vi "XNET CAN Signal Logger - MultiPorts.vi"() -> ()   [LabVIEW 2021, in "XNET-CAN-Signal-Logger.lvlib"]
uses:
  XNET-CAN-Signal-Logger.lvlib
  Typedef/Def-CAN Port Configuration.ctl
  Typedef/Def-Data Queue Ref.ctl
  Typedef/Def-Data Queue Type.ctl
  SubVIs/Global Variables.vi
  <resource>/objmgr/xnet.rc
panel:
  out "State:":string
  in  "Tab Control":enum32{"Analog Input", "CAN"}(tab)=enum."CAN"
  in  "CAN Configurations":T1[](array[typedef]) {"Sample Rate (Hz)" format="%#_13g"}
  in  "Stop Logging":bool
  out "Monitor.SignalUnits":string[](array[string])
  out "Monitor.SignalValues":dbl[](array[numeric])
  in  "Monitor.SignalNames":string[](array[combo])
  out "# elements in queue:":i32
  in  "Start Logging":bool
  out "Preview:":string
  in  "Log file name":string="LogFile_{Year}-{Month}-{Day}-{Hour}-{Minute}-{Second}.tdms"
  in  "Log file folder":path=path "C:/Users/NI/Desktop/Data"
  in  "Exit":bool
  # "Configuration"
  # "Signals to Monitor"
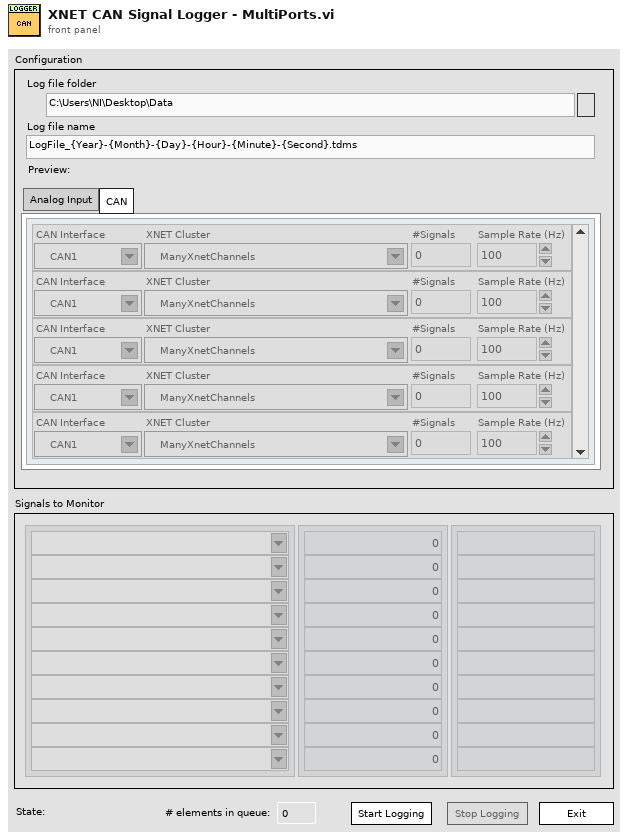
[diagram p1: front panel]
types:
  T1 = typedef "XNET-CAN-Signal-Logger.lvlib/Def-CAN Port Configuration.ctl" = cluster{"CAN Interface":refnum<k21>, "XNET Cluster":refnum<k21>, "#Signals":i32, "Sample Rate (Hz)":dbl}
  T2 = enum32{"Invalid", "Standard", "Closed", "Hidden", "Minimized", "Maximized"}
  T3 = enum32{"invalid app kind", "Development System", "Run Time System", "Student Edition", "Embedded LabVIEW", "Evaluation", "Custom"}
  T4 = enum8{"Enabled", "Disabled", "Disabled and Grayed Out"}
  T5 = typedef "XNET-CAN-Signal-Logger.lvlib/Def-Data Queue Type.ctl" = cluster{"PackageID":i32, "Data":waveform(dbl)[]}
  T6 = typedef "XNET-CAN-Signal-Logger.lvlib/Def-Data Queue Ref.ctl" = refnum<queue>
  T7 = cluster{"Core":cluster{"Current VI Reference":refnum<vi>, "Close Panel on Exit?":bool}, "Logging State":enum16{"Configure", "Logging"}, "LogFilePath":path, "CAN Configurations":refnum<vi>, "Data Queue Ref":T6, "Error Queue Ref":refnum<queue>, "Monitor.SignalNames":string[], "Monitor.SignalUnits":string[]}
  T8 = cluster{"Current VI Reference":refnum<vi>, "Close Panel on Exit?":bool}
  T9 = typedef "Def-CAN Port Configuration.ctl" = cluster{"CAN Interface":refnum<k21>, "XNET Cluster":refnum<k21>, "#Signals":i32, "Sample Rate (Hz)":dbl}
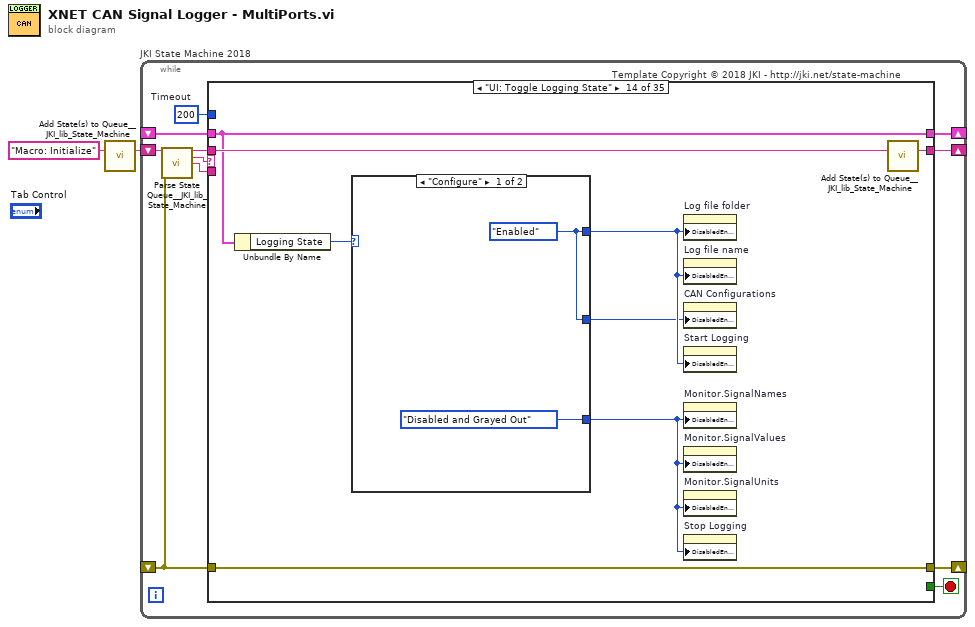
[diagram p0: block diagram]
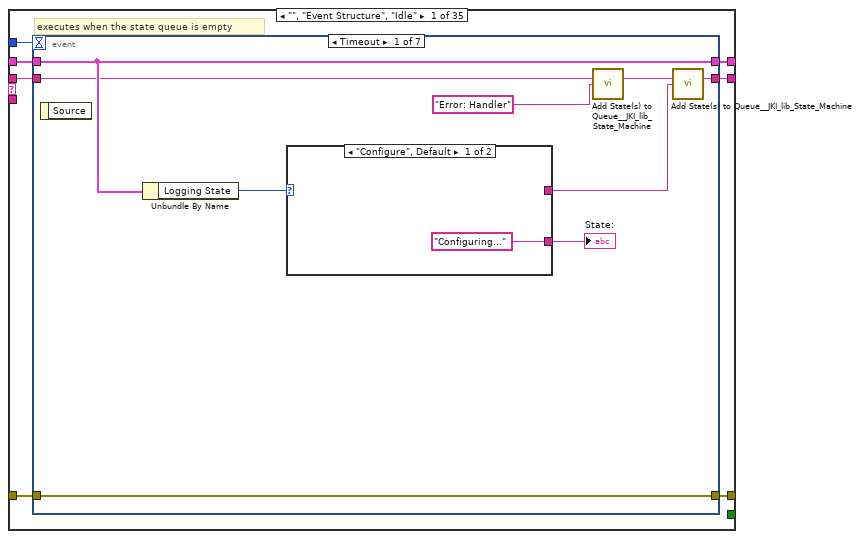
[diagram p2: hidden frame]
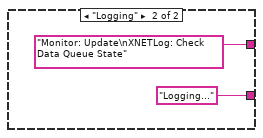
[diagram p3: hidden frame]
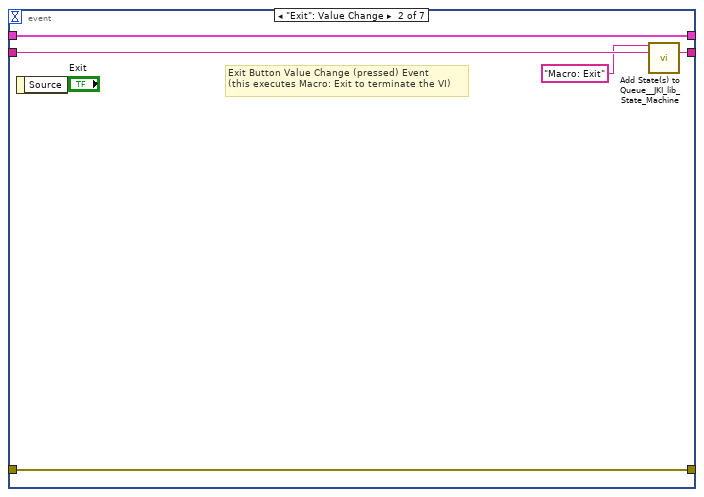
[diagram p4: hidden frame]
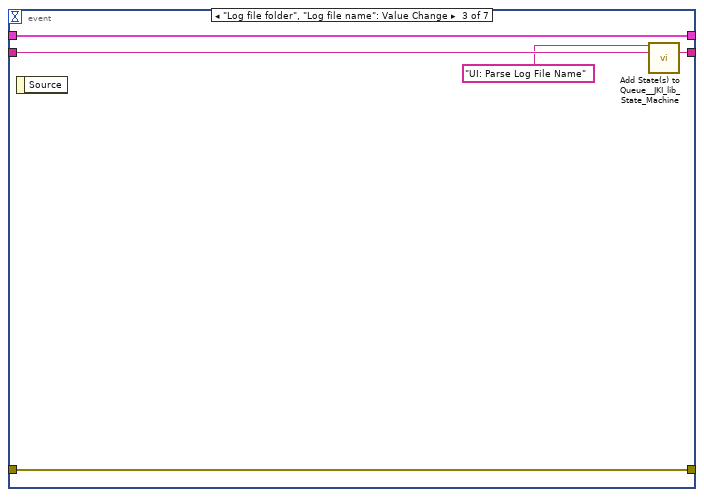
[diagram p5: hidden frame]
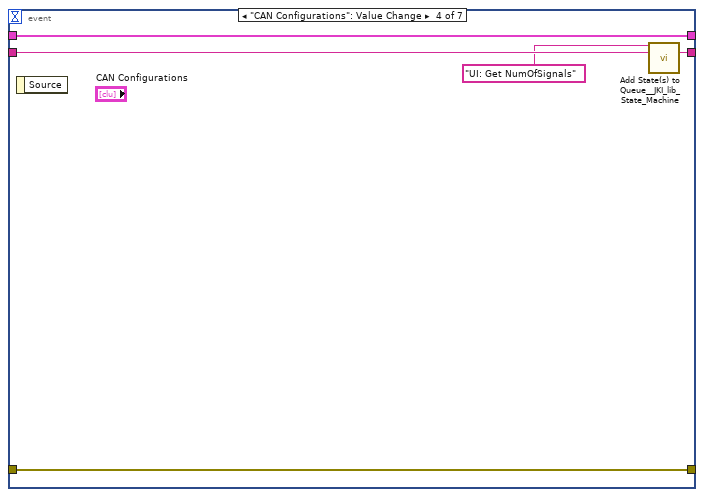
[diagram p6: hidden frame]
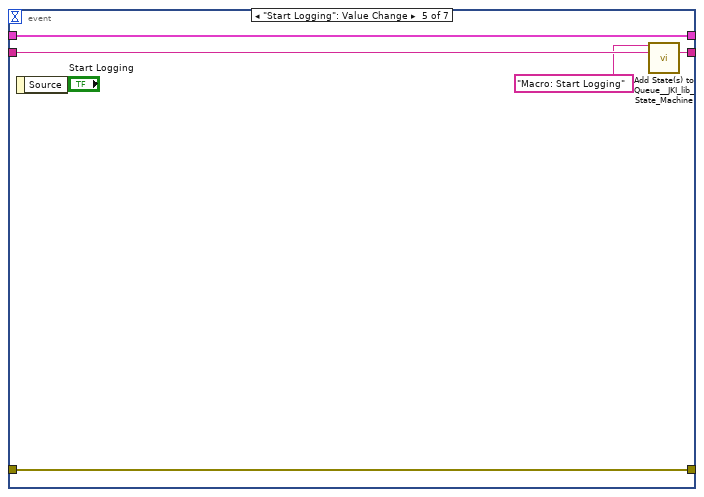
[diagram p7: hidden frame]
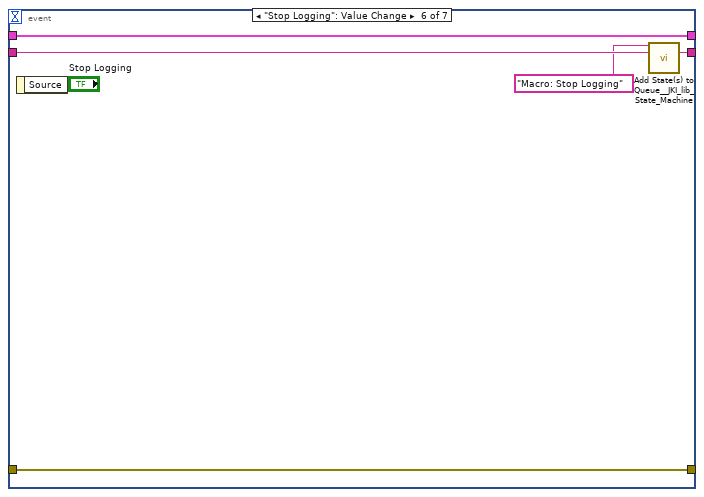
[diagram p8: hidden frame]
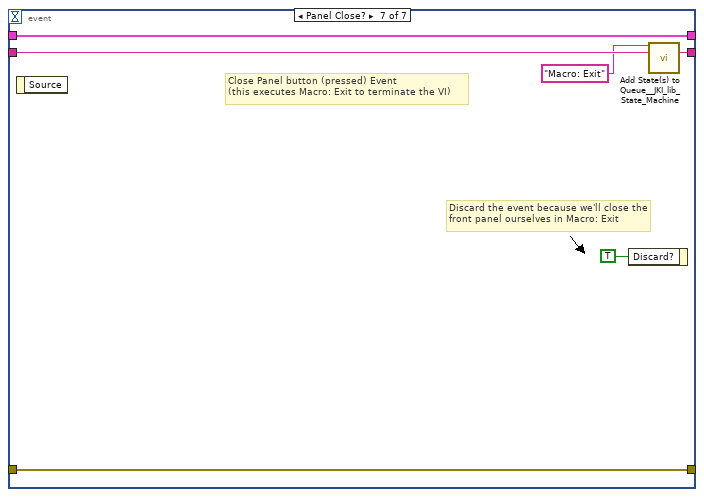
[diagram p9: hidden frame]
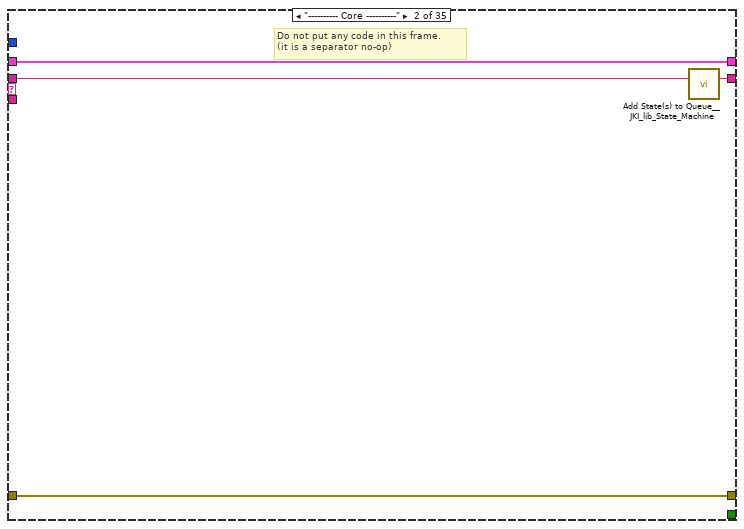
[diagram p10: hidden frame]
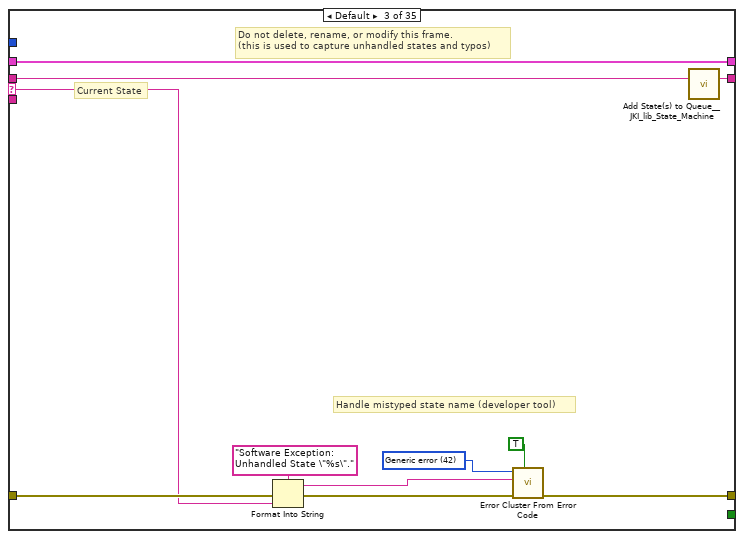
[diagram p11: hidden frame]
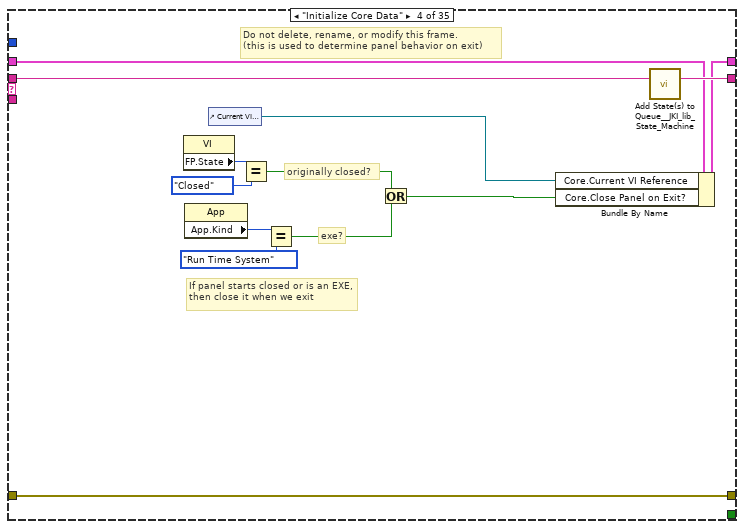
[diagram p12: hidden frame]
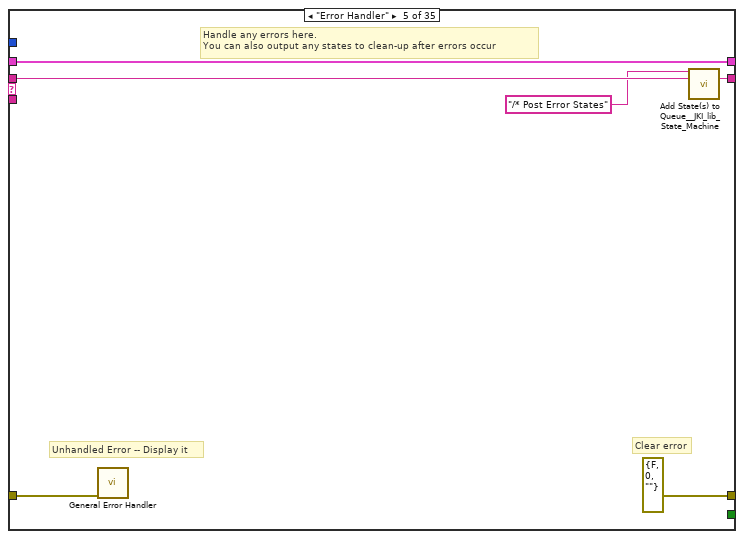
[diagram p13: hidden frame]
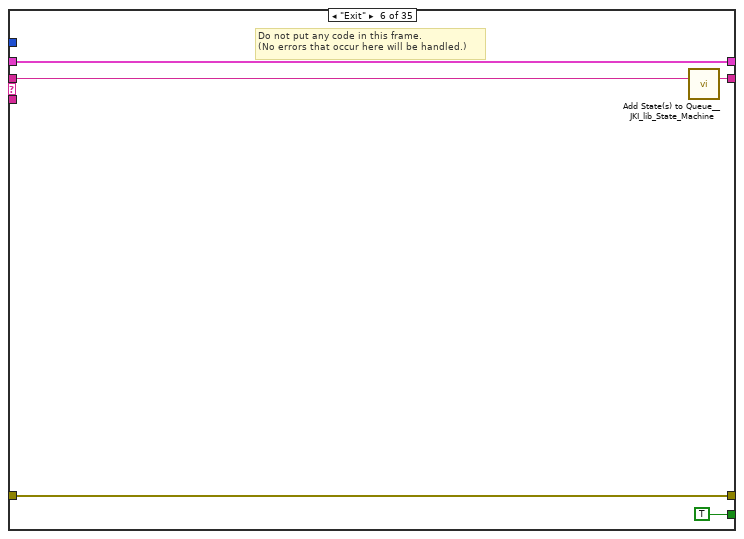
[diagram p14: hidden frame]
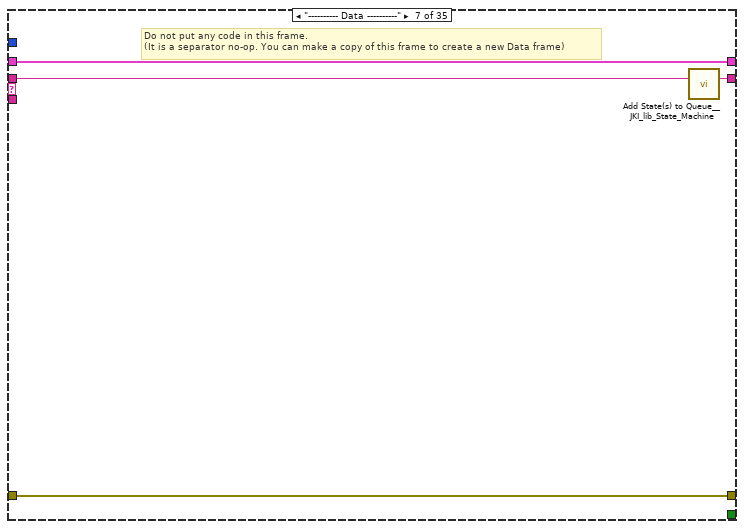
[diagram p15: hidden frame]
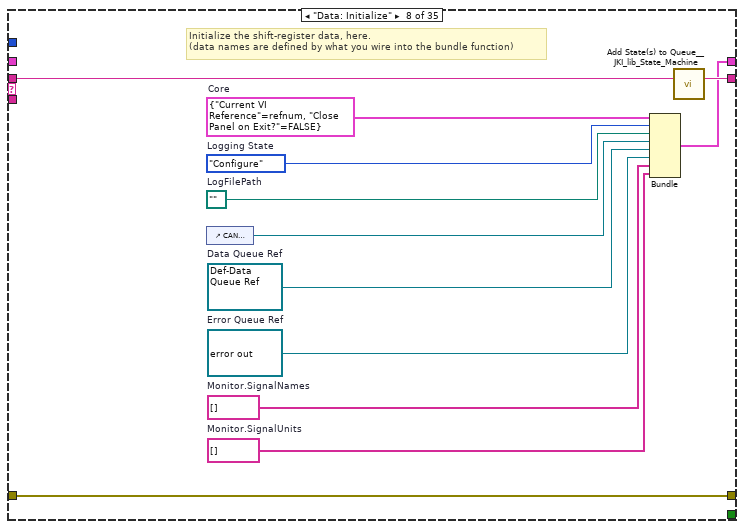
[diagram p16: hidden frame]
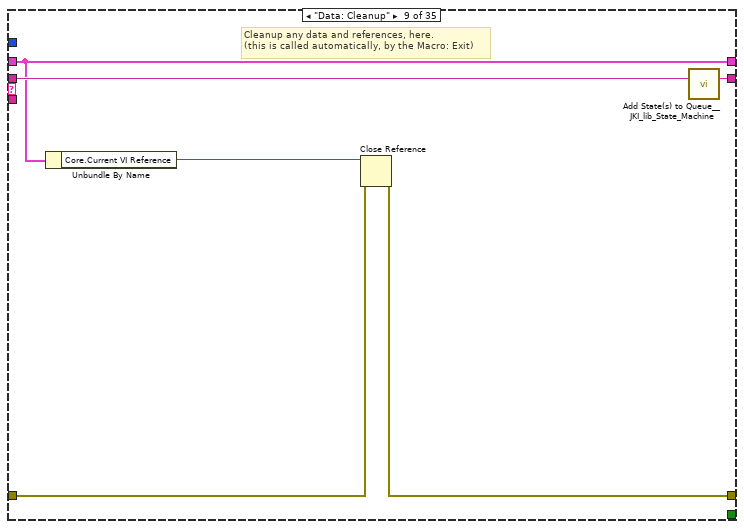
[diagram p17: hidden frame]
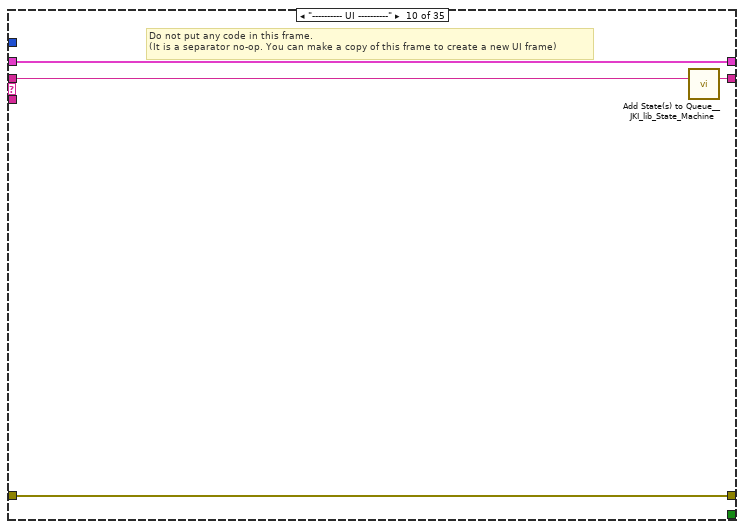
[diagram p18: hidden frame]
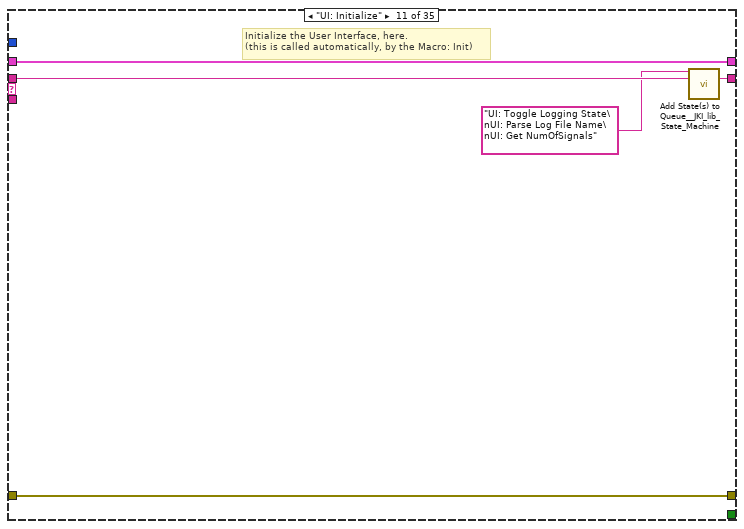
[diagram p19: hidden frame]
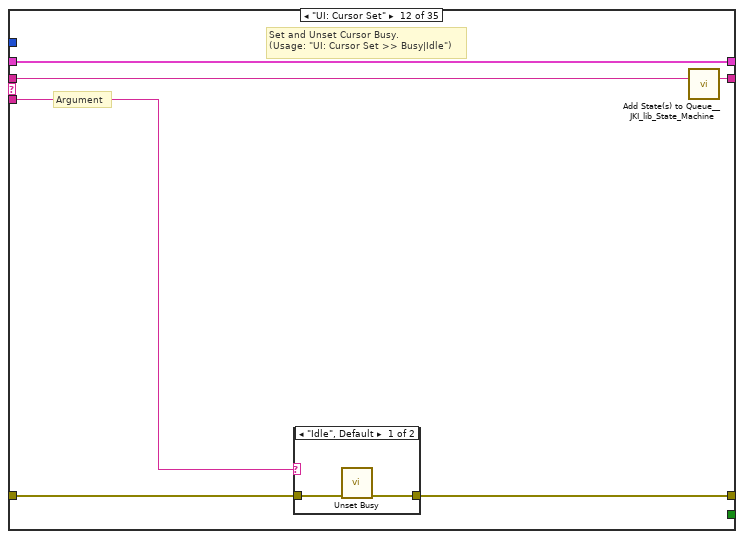
[diagram p20: hidden frame]
diagram:
  n1 = call <vilib>:"Add State(s) to Queue__JKI_lib_State_Machine.vi"("State(s) in (\"\")"="Macro: Initialize") -> ("States Out"=w2:string)  [unwired: 14 in]
  n2 = while "JKI State Machine 2018" {
    shift-right: [w6] -> _
    shift-left: _ -> [w5]
    shift-right: [w9] -> _
    shift-left: _ -> [w3]
    shift-right: [w8] -> _
    shift-left: w2 -> [w10]
    stop <- w7 stop-if-true
    w4 = 200  # Timeout
    # "Template Copyright © 2018 JKI - http://jki.net/state-machine"
    n3 = call <vilib>:"Parse State Queue__JKI_lib_State_Machine.vi"("State Queue"=w10, "Error In (no error)"=w3) -> ("Remaining States"=w12:string, "Current State"=w13:string, "Arguments"=w11:string)  [unwired: 11 in]
    n4 = case shown="\"UI: Toggle Logging State\"" w13 {
      selector: w13 -> [_ _ w68 _ _ _ _ _ _ _ _ _ _ _ _ _ _ _ _ _ _ _ _ _ _ _ _ _ _ _ _ _ _ _ _]
      tunnel: w12 -> [w20 w67 w72 w91 w97 w102 w106 w118 w124 w128 w133 w139 w150 w223 w237 w245 w254 w259 w266 w273 w283 w287 w295 w301 w310 w314 w323 w329 w336 w344 w351 w357 w362 w377 w388]
      tunnel: w11 -> [_ _ _ _ _ _ _ _ _ _ _ w134 w144 _ _ _ _ _ _ _ _ _ _ _ _ _ _ _ _ _ _ w353 _ _ _]
      tunnel: w5 -> [w18 w64 w70 w84 w94 w100 w103 _ w119 w125 w131 w137 w146 w220 w234 w242 w251 w256 w263 w270 w280 w284 w293 w299 w308 w311 w321 w327 w334 w342 w349 w354 w359 w374 w384]
      tunnel: [w17 w65 w74 w88 errorcluster {"status"=FALSE, "code"=0, "source"=""} ("error out") w99 w104 w115 w120 w126 w130 w135 w147 w221 w235 w243 w252 w257 w264 w271 w281 w285 w291 w296 w303 w312 w317 w324 w331 w339 w347 w355 w360 w363 w385] -> w9
      tunnel: w3 -> [w16 w65 w73 w88 w93 w99 w104 w115 w121 w126 w130 w136 w148 w221 w235 w243 w252 w257 w264 w271 w281 w285 w289 w297 w306 w312 w318 w325 w332 w340 w348 w355 w360 w370 w386]
      tunnel: [w19 w66 w71 w90 w96 w101 w105 w117 w123 w127 w132 w138 w149 w222 w236 w244 w253 w258 w265 w272 w282 w286 w294 w300 w309 w313 w322 w328 w335 w343 w350 w356 w361 w376 w387] -> w8
      tunnel: [_ _ _ _ _ TRUE _ _ _ _ _ _ _ _ _ _ _ _ _ _ _ _ _ _ _ _ _ _ _ _ _ _ _ _ _] -> w7
      tunnel: [w15 w64 w70 w89 w94 w100 w103 w116 w119 w125 w131 w137 w146 w220 w230 w242 w251 w256 w261 w268 w280 w284 w290 w299 w308 w311 w316 w327 w334 w342 w349 w354 w359 w371 w384] -> w6
      tunnel: w4 -> [w14 _ _ _ _ _ _ _ _ _ _ _ _ _ _ _ _ _ _ _ _ _ _ _ _ _ _ _ _ _ _ _ _ _ _]
      frame "", "Event Structure", "Idle" {
        # "executes when the state queue is empty"
        n5 = event shown="[0] Timeout" {
          selector: _ -> [_ _ _ _ _ _ _]
          dyn-events: _ -> [_ _ _ _ _ _ _]
          timeout: w14 -> [_ _ _ _ _ _ _]
          tunnel: w20 -> [w24 w37 w42 w47 w52 w57 w63]
          tunnel: [w29 w36 w41 w46 w51 w56 w62] -> w19
          tunnel: w18 -> [w27 w34 w39 w44 w48 w53 w60]
          tunnel: [w28 w35 w40 w45 w50 w55 w61] -> w17
          tunnel: w16 -> [w28 w35 w40 w45 w50 w55 w61]
          tunnel: [w27 w34 w39 w44 w48 w53 w60] -> w15
          event Timeout {
            n6 = event-data() -> ()  [unwired: 1 in, 1 out]
            n7 = Unbundle By Name(w27) -> ("Logging State"=w26:enum16{"Configure", "Logging"})
            n8 = case shown="\"Configure\", Default" w26 {
              tunnel: [_ "Monitor: Update\nXNETLog: Check Data Queue State" ("State(s) at Back (\"\")")] -> w22
              tunnel: ["Configuring..." ("State:") "Logging..." ("State:")] -> w21
              frame "Configure", Default {
              }
              frame "Logging" {
              }
            }
            "State:" <- w21
            n9 = call <vilib>:"Add State(s) to Queue__JKI_lib_State_Machine.vi"("State(s) in (\"\")"=w24, "State(s) at Back (\"\")"="Error: Handler" ("string")) -> ("States Out"=w23:string)  [unwired: 13 in]
            n10 = call <vilib>:"Add State(s) to Queue__JKI_lib_State_Machine.vi"("State(s) in (\"\")"=w23, "State(s) at Back (\"\")"=w22) -> ("States Out"=w29:string)  [unwired: 13 in]
          }
          event "Exit": Value Change {
            # "Exit Button Value Change (pressed) Event\n(this executes Macro: Exit to terminate the VI)"
            n11 = event-data() -> ()  [unwired: 1 in, 1 out]
            n12 = call <vilib>:"Add State(s) to Queue__JKI_lib_State_Machine.vi"("State(s) in Front (\"\")"="Macro: Exit", "State(s) in (\"\")"=w37) -> ("States Out"=w36:string)  [unwired: 13 in]
          }
          event "Log file folder", "Log file name": Value Change {
            n13 = event-data() -> ()  [unwired: 1 in, 1 out]
            n14 = call <vilib>:"Add State(s) to Queue__JKI_lib_State_Machine.vi"("State(s) in Front (\"\")"="UI: Parse Log File Name", "State(s) in (\"\")"=w42) -> ("States Out"=w41:string)  [unwired: 13 in]
          }
          event "CAN Configurations": Value Change {
            n15 = event-data() -> ()  [unwired: 1 in, 1 out]
            n16 = call <vilib>:"Add State(s) to Queue__JKI_lib_State_Machine.vi"("State(s) in Front (\"\")"="UI: Get NumOfSignals", "State(s) in (\"\")"=w47) -> ("States Out"=w46:string)  [unwired: 13 in]
          }
          event "Start Logging": Value Change {
            n17 = event-data() -> ()  [unwired: 1 in, 1 out]
            n18 = call <vilib>:"Add State(s) to Queue__JKI_lib_State_Machine.vi"("State(s) in Front (\"\")"="Macro: Start Logging", "State(s) in (\"\")"=w52) -> ("States Out"=w51:string)  [unwired: 13 in]
          }
          event "Stop Logging": Value Change {
            n19 = event-data() -> ()  [unwired: 1 in, 1 out]
            n20 = call <vilib>:"Add State(s) to Queue__JKI_lib_State_Machine.vi"("State(s) in Front (\"\")"="Macro: Stop Logging", "State(s) in (\"\")"=w57) -> ("States Out"=w56:string)  [unwired: 13 in]
          }
          event Panel Close? {
            # "Discard the event because we'll close the front panel ourselves in Macro: Exit"
            # "Close Panel button (pressed) Event\n(this executes Macro: Exit to terminate the VI)"
            n21 = event-data() -> ()  [unwired: 1 in, 1 out]
            n22 = event-data("Discard?"=TRUE) -> ()  [unwired: 1 in, 1 out]
            n23 = call <vilib>:"Add State(s) to Queue__JKI_lib_State_Machine.vi"("State(s) in Front (\"\")"="Macro: Exit", "State(s) in (\"\")"=w63) -> ("States Out"=w62:string)  [unwired: 13 in]
          }
        }
      }
      frame "---------- Core ----------" {
        # "Do not put any code in this frame.\n(it is a separator no-op)"
        n24 = call <vilib>:"Add State(s) to Queue__JKI_lib_State_Machine.vi"("State(s) in (\"\")"=w67) -> ("States Out"=w66:string)  [unwired: 14 in]
      }
      frame Default {
        w77 = 42 items=["No error", "Argument error", "Memory is full", "Out of zone", "End of file", "File already open", "Generic file I/O error", "File not found", "File permission error", "Disk is full", "Duplicate path", "Too many files open", "System feature not enabled", "Resource file not found", "Cannot add resource", "Resource not found", "Image not found", "Image memory error", "Pen does not exist", "Config type invalid", "Config token not found", "Config parse error", "Config memory error", "Bad external code format", "Bad external code offset", "External code not present", "Null window", "Destroy window error", "Null menu", "Print aborted", "Bad print record", "Print driver error", "Windows error during printing", "Memory error during printing", "Print dialog error", "Generic print error", "Invalid device refnum", "Device not found", "Device parameter error", "Device unit error", "Cannot open device", "Device call aborted", "Generic error", "Cancelled by user", "Object ID too low", "Object ID too high", "Object not in heap", "Unknown heap", "Unknown object (invalid DefProc)", "Unknown object (DefProc not in table)", "Message out of range", "Invalid (null) method", "Unknown message", "Manager call not supported", "Bad address", "Network operation in progress", "Network operation timed out", "Connection is busy", "Network attribute not supported", "Network error", "Address in use", "System out of memory", "Connection aborted", "Connection refused", "Not connected", "Already connected", "Connection closed", "Initialization error (interapplication manager)", "Bad occurrence", "Wait on unbound occurrence handler", "Occurrence queue overflow", "Datalog type conflict", "Unused", "Unrecognized type (interapplication manager)", "Memory corrupt", "Failed to make temporary DLL", "Old CIN version", "Drag socket not found", "Failed to load drop-object", "Failed to register OLE object", "Failed to release OLE object", "Format specifier type mismatch", "Unknown format specifier", "Too few format specifiers", "Too many format specifiers", "Scan failed", "Newer CIN version", "Error converting to variant", "Runtime menu error", "Password tampered", "Variant attribute not found", "Incompatible variant data type", "Event data is not available", "Event Store is not present", "Occurrence is not found", "Event Queue is not created", "Event info is not available", "Refnum passed is NULL", "Error retrieving Class GUID", "Error retrieving CoClass GUID", "Error retrieving TypeLib GUID.", "Bad built application magic bytes.", "Specific driver is different from the specific driver associated with the Logical Name.", "There is no session opened to the class driver.", "Max Error", "MAX - Error with config objects", "MAX - Error loading configuration", "MAX - Group not supported"]
        # "Current State"
        # "Do not delete, rename, or modify this frame.\n(this is used to capture unhandled states and typos)"
        # "Handle mistyped state name (developer tool)"
        n25 = Format Into String(format string="Software Exception: Unhandled State \"%s\"." ("message"), error in=w73, w68) -> (resulting string=w76:string, error out=w75:errorcluster)  [unwired: 1 in]
        n26 = call <vilib>:"Error Cluster From Error Code.vi"("show call chain? (False)"=TRUE, "error in (no error)"=w75, "error message (\"\")"=w76, "error code (0)"=w77) -> ("error out"=w74:errorcluster)  [unwired: 5 in]
        n27 = call <vilib>:"Add State(s) to Queue__JKI_lib_State_Machine.vi"("State(s) in (\"\")"=w72) -> ("States Out"=w71:string)  [unwired: 14 in]
      }
      frame "Initialize Core Data" {
        # "Do not delete, rename, or modify this frame.\n(this is used to determine panel behavior on exit)"
        # "originally closed?"
        # "exe?"
        # "If panel starts closed or is an EXE, then close it when we exit"
        n28 = property class="VI"() -> ("FP.State"=w81:T2)  [unwired: 2 in, 2 out]
        n29 = property class="App"() -> ("App.Kind"=w87:T3)  [unwired: 2 in, 2 out]
        n30 = control-ref of="Current VI Reference"() -> (w82:refnum<vi>)
        n31 = Equal?(x=w81, y=T2."Closed" ("Front Panel Window:State")) -> (x = y?=w79:bool)
        n32 = Equal?(x=w87, y=T3."Run Time System" ("Application:Kind")) -> (x = y?=w85:bool)
        n33 = Or(x=w79, y=w85) -> (x .or. y?=w83:bool)
        n34 = Bundle By Name(cluster=w84, "Core.Current VI Reference"=w82, "Core.Close Panel on Exit?"=w83) -> (w89:T7)
        n35 = call <vilib>:"Add State(s) to Queue__JKI_lib_State_Machine.vi"("State(s) in (\"\")"=w91) -> ("States Out"=w90:string)  [unwired: 14 in]
      }
      frame "Error Handler" {
        # "Unhandled Error -- Display it"
        # "Handle any errors here.\nYou can also output any states to clean-up after errors occur"
        # "Clear error"
        n36 = call <vilib>:"General Error Handler.vi"("error in (no error)"=w93) -> ()  [unwired: 10 in, 5 out]
        n37 = call <vilib>:"Add State(s) to Queue__JKI_lib_State_Machine.vi"("State(s) in Front (\"\")"="/* Post Error States", "State(s) in (\"\")"=w97) -> ("States Out"=w96:string)  [unwired: 13 in]
      }
      frame "Exit" {
        # "Do not put any code in this frame.\n(No errors that occur here will be handled.)"
        n38 = call <vilib>:"Add State(s) to Queue__JKI_lib_State_Machine.vi"("State(s) in (\"\")"=w102) -> ("States Out"=w101:string)  [unwired: 14 in]
      }
      frame "---------- Data ----------" {
        # "Do not put any code in this frame.\n(It is a separator no-op. You can make a copy of this frame to create a new Data frame)"
        n39 = call <vilib>:"Add State(s) to Queue__JKI_lib_State_Machine.vi"("State(s) in (\"\")"=w106) -> ("States Out"=w105:string)  [unwired: 14 in]
      }
      frame "Data: Initialize" {
        w108 = string[] []  # Monitor.SignalUnits
        w107 = string[] []  # Monitor.SignalNames
        w109 = refnum<queue> refnum  # Error Queue Ref
        w110 = T6 refnum  # Data Queue Ref
        w111 = enum16{"Configure", "Logging"}."Configure"  # Logging State
        w113 = path ""  # LogFilePath
        w114 = T8 {"Current VI Reference"=refnum, "Close Panel on Exit?"=FALSE}  # Core
        # "Initialize the shift-register data, here.\n(data names are defined by what you wire into the bundle function)"
        n40 = control-ref of="CAN Configurations"() -> (w112:refnum<vi>)
        n41 = Bundle("Core"=w114, "Logging State"=w111, "LogFilePath"=w113, "CAN Configurations"=w112, "Data Queue Ref"=w110, "Error Queue Ref"=w109, "Monitor.SignalNames"=w107, "Monitor.SignalUnits"=w108) -> (w116:T7)  [unwired: 1 in]
        n42 = call <vilib>:"Add State(s) to Queue__JKI_lib_State_Machine.vi"("State(s) in (\"\")"=w118) -> ("States Out"=w117:string)  [unwired: 14 in]
      }
      frame "Data: Cleanup" {
        # "Cleanup any data and references, here.\n(this is called automatically, by the Macro: Exit)"
        n43 = Unbundle By Name(w119) -> ("Core.Current VI Reference"=w122:refnum<vi>)
        n44 = Close Reference(reference=w122, error in (no error)=w121) -> (error out=w120:errorcluster)
        n45 = call <vilib>:"Add State(s) to Queue__JKI_lib_State_Machine.vi"("State(s) in (\"\")"=w124) -> ("States Out"=w123:string)  [unwired: 14 in]
      }
      frame "---------- UI ----------" {
        # "Do not put any code in this frame.\n(It is a separator no-op. You can make a copy of this frame to create a new UI frame)"
        n46 = call <vilib>:"Add State(s) to Queue__JKI_lib_State_Machine.vi"("State(s) in (\"\")"=w128) -> ("States Out"=w127:string)  [unwired: 14 in]
      }
      frame "UI: Initialize" {
        # "Initialize the User Interface, here.\n(this is called automatically, by the Macro: Init)"
        n47 = call <vilib>:"Add State(s) to Queue__JKI_lib_State_Machine.vi"("State(s) in Front (\"\")"="UI: Toggle Logging State\nUI: Parse Log File Name\nUI: Get NumOfSignals" ("State(s) in Front (\"\")"), "State(s) in (\"\")"=w133) -> ("States Out"=w132:string)  [unwired: 13 in]
      }
      frame "UI: Cursor Set" {
        # "Argument"
        # "Set and Unset Cursor Busy.\n(Usage: \"UI: Cursor Set >> Busy|Idle\")"
        n48 = case shown="\"Idle\", Default" w134 {
          tunnel: w136 -> [w141 w143]
          tunnel: [w140 w142] -> w135
          frame "Idle", Default {
            n49 = call <vilib>:"Unset Busy.vi"("error in (no error)"=w141) -> ("error out"=w140:errorcluster)  [unwired: 10 in]
          }
          frame "Busy" {
            n50 = call <vilib>:"Set Busy.vi"("error in (no error)"=w143) -> ("error out"=w142:errorcluster)  [unwired: 9 in, 1 out]
          }
        }
        n51 = call <vilib>:"Add State(s) to Queue__JKI_lib_State_Machine.vi"("State(s) in (\"\")"=w139) -> ("States Out"=w138:string)  [unwired: 14 in]
      }
      frame "UI: Front Panel State" {
        # "Argument"
        # "Set Front Panel Open or Closed\n(Usage: \"UI: Front Panel State >> Open|Close\")"
        n52 = Unbundle By Name(w146) -> ("Core.Current VI Reference"=w145:refnum<vi>)
        n53 = case shown="\"Minimize\", \"Minimized\"" w144 {
          tunnel: w148 -> [w156 w171 w182 w195 w208]
          tunnel: [w158 w172 w184 w197 w210] -> w147
          tunnel: w145 -> [w157 w169 w183 w196 w209]
          frame "Open", "Standard", Default {
            w151 = T2."Standard" ("State")
            n54 = property class="VI"(reference=w157, error in=w156) -> (reference out=w154:refnum<vi>, error out=w155:errorcluster, "FP.State"=w153:T2)
            n55 = Not Equal?(x=w153, y=w151) -> (x != y?=w152:bool)
            n56 = case shown="True" w152 {
              tunnel: [w162 w164] -> w158
              tunnel: w155 -> [w161 w164]
              tunnel: w154 -> [w160 _]
              tunnel: w151 -> [w159 _]
              frame True {
                n57 = invoke class="VI" method="FP.Open"(reference=w160, error in=w161, "Activate"=TRUE, "State"=w159) -> (error out=w162:errorcluster)  [unwired: 1 in, 4 out]
              }
              frame False {
              }
            }
          }
          frame "Close", "Closed" {
            n58 = property class="VI"(reference=w169, error in=w171) -> (reference out=w168:refnum<vi>, error out=w170:errorcluster, "FP.State"=w166:T2)
            n59 = Not Equal?(x=w166, y=T2."Closed" ("Front Panel Window:State")) -> (x != y?=w165:bool)
            n60 = case shown="True" w165 {
              tunnel: [w173 w176] -> w172
              tunnel: w170 -> [w173 w175]
              tunnel: w168 -> [_ w174]
              frame False {
              }
              frame True {
                n61 = invoke class="VI" method="FP.Close"(reference=w174, error in=w175) -> (error out=w176:errorcluster)  [unwired: 1 in, 2 out]
              }
            }
          }
          frame "Hidden", "Hide" {
            w177 = T2."Hidden" ("State")
            n62 = property class="VI"(reference=w183, error in=w182) -> (reference out=w180:refnum<vi>, error out=w181:errorcluster, "FP.State"=w179:T2)
            n63 = Not Equal?(x=w179, y=w177) -> (x != y?=w178:bool)
            n64 = case shown="True" w178 {
              tunnel: [w188 w189] -> w184
              tunnel: w181 -> [w187 w189]
              tunnel: w180 -> [w186 _]
              tunnel: w177 -> [w185 _]
              frame True {
                n65 = invoke class="VI" method="FP.Open"(reference=w186, error in=w187, "State"=w185) -> (error out=w188:errorcluster)  [unwired: 2 in, 4 out]
              }
              frame False {
              }
            }
          }
          frame "Minimize", "Minimized" {
            w190 = T2."Minimized" ("State")
            n66 = property class="VI"(reference=w196, error in=w195) -> (reference out=w193:refnum<vi>, error out=w194:errorcluster, "FP.State"=w192:T2)
            n67 = Not Equal?(x=w192, y=w190) -> (x != y?=w191:bool)
            n68 = case shown="True" w191 {
              tunnel: [w201 w202] -> w197
              tunnel: w194 -> [w200 w202]
              tunnel: w193 -> [w199 _]
              tunnel: w190 -> [w198 _]
              frame True {
                n69 = invoke class="VI" method="FP.Open"(reference=w199, error in=w200, "State"=w198) -> (error out=w201:errorcluster)  [unwired: 2 in, 4 out]
              }
              frame False {
              }
            }
          }
          frame "Maximize", "Maximized" {
            w203 = T2."Maximized" ("State")
            n70 = property class="VI"(reference=w209, error in=w208) -> (reference out=w206:refnum<vi>, error out=w207:errorcluster, "FP.State"=w205:T2)
            n71 = Not Equal?(x=w205, y=w203) -> (x != y?=w204:bool)
            n72 = case shown="True" w204 {
              tunnel: [w214 w215] -> w210
              tunnel: w207 -> [w213 w215]
              tunnel: w206 -> [w212 _]
              tunnel: w203 -> [w211 _]
              frame True {
                n73 = invoke class="VI" method="FP.Open"(reference=w212, error in=w213, "State"=w211) -> (error out=w214:errorcluster)  [unwired: 2 in, 4 out]
              }
              frame False {
              }
            }
          }
        }
        n74 = call <vilib>:"Add State(s) to Queue__JKI_lib_State_Machine.vi"("State(s) in (\"\")"=w150) -> ("States Out"=w149:string)  [unwired: 14 in]
      }
      frame "UI: Toggle Logging State" {
        n75 = Unbundle By Name(w220) -> ("Logging State"=w219:enum16{"Configure", "Logging"})
        n76 = case shown="\"Configure\"" w219 {
          tunnel: [w224 T4."Disabled and Grayed Out" ("Disabled")] -> w218
          tunnel: [T4."Disabled and Grayed Out" ("Disabled") T4."Enabled" ("Disabled")] -> w217
          tunnel: [w224 T4."Disabled" ("Disabled")] -> w216
          frame "Configure" {
            w224 = T4."Enabled" ("Disabled")
          }
          frame "Logging" {
          }
        }
        n77 = property on="Log file folder" class="Path"("DisabledEnum"=w218) -> ()  [unwired: 2 in, 2 out]
        n78 = property on="Log file name" class="Str"("DisabledEnum"=w218) -> ()  [unwired: 2 in, 2 out]
        n79 = property on="CAN Configurations" class="Arr (strict)"("DisabledEnum"=w216) -> ()  [unwired: 2 in, 2 out]
        n80 = property on="Start Logging" class="Bool"("DisabledEnum"=w218) -> ()  [unwired: 2 in, 2 out]
        n81 = property on="Monitor.SignalNames" class="Arr (strict)"("DisabledEnum"=w217) -> ()  [unwired: 2 in, 2 out]
        n82 = property on="Monitor.SignalValues" class="Arr (strict)"("DisabledEnum"=w217) -> ()  [unwired: 2 in, 2 out]
        n83 = property on="Monitor.SignalUnits" class="Arr (strict)"("DisabledEnum"=w217) -> ()  [unwired: 2 in, 2 out]
        n84 = property on="Stop Logging" class="Bool"("DisabledEnum"=w217) -> ()  [unwired: 2 in, 2 out]
        n85 = call <vilib>:"Add State(s) to Queue__JKI_lib_State_Machine.vi"("State(s) in (\"\")"=w223) -> ("States Out"=w222:string)  [unwired: 14 in]
      }
      frame "UI: Parse Log File Name" {
        n86 = call "Parse Log File Name.vi"("Log file name"="Log file name") -> ("Parsed Log file name"=w232:string)  [unwired: 10 in]
        "Preview:" <- w232
        n87 = Build Path(base path="Log file folder", name or relative path=w232) -> (appended path=w229:path)
        n88 = Bundle By Name(cluster=w234, "LogFilePath"=w229) -> (w230:T7)
        n89 = call <vilib>:"Add State(s) to Queue__JKI_lib_State_Machine.vi"("State(s) in (\"\")"=w237) -> ("States Out"=w236:string)  [unwired: 14 in]
      }
      frame "UI: Get NumOfSignals" {
        n90 = Unbundle By Name(w242) -> ("CAN Configurations"=w241:refnum<vi>)
        n91 = property class="Arr (strict)"(reference=w241) -> (reference out=w239:refnum<vi>, "Value"=w240:T9[])  [unwired: 1 in, 1 out]
        n92 = for {
          tunnel: w240 -> [w248] mode=indexing
          tunnel: [w246] -> w238 mode=indexing
          n93 = Unbundle By Name(w248) -> ("XNET Cluster"=w250:refnum<k21>)
          n94 = property class="XNET Cluster"(reference=w250) -> ("Sigs"=w249:refnum<k21>[])  [unwired: 1 in, 2 out]
          n95 = Array Size(array=w249) -> (size(s)=w247:i32)
          n96 = Bundle By Name(cluster=w248, "#Signals"=w247) -> (w246:T9)
        }
        n97 = property class="Arr (strict)"(reference=w239, "Value"=w238) -> ()  [unwired: 1 in, 2 out]
        n98 = call <vilib>:"Add State(s) to Queue__JKI_lib_State_Machine.vi"("State(s) in (\"\")"=w245) -> ("States Out"=w244:string)  [unwired: 14 in]
      }
      frame "---------- Macro ----------" {
        # "Do not put any code in this frame.\n(It is a separator no-op. You can make a copy of this frame to create a new Macro frame)"
        n99 = call <vilib>:"Add State(s) to Queue__JKI_lib_State_Machine.vi"("State(s) in (\"\")"=w254) -> ("States Out"=w253:string)  [unwired: 14 in]
      }
      frame "Macro: Initialize" {
        w255 = "Data: Initialize\nInitialize Core Data\n\nError: Obtain Error Queue\n\nUI: Initialize\nUI: Front Panel State >> Open"  # Data: Initialize Initialize Core Data  Error: Obtain Error Queue  UI: Initialize UI: Front Panel State >> Open
        # "Initialization Macro\n(This is called once, when the VI starts)"
        n100 = call <vilib>:"Add State(s) to Queue__JKI_lib_State_Machine.vi"("State(s) in Front (\"\")"=w255, "State(s) in (\"\")"=w259) -> ("States Out"=w258:string)  [unwired: 13 in]
      }
      frame "Macro: Start Logging" {
        n101 = Bundle By Name(cluster=w263, "Logging State"=enum16{"Configure", "Logging"}."Logging") -> (w261:T7)
        n102 = call <vilib>:"Add State(s) to Queue__JKI_lib_State_Machine.vi"("State(s) in Front (\"\")"="UI: Toggle Logging State\nUI: Parse Log File Name\nXNETLog: Obtain Data Queue\nXNETLog: Global Stop >> FALSE\nXNETLog: Launch TDMS Writer\nXNETLog: Launch XNET CAN Reader\nMonitor: Initialize" ("State(s) in Front (\"\")"), "State(s) in (\"\")"=w266) -> ("States Out"=w265:string)  [unwired: 13 in]
      }
      frame "Macro: Stop Logging" {
        n103 = Bundle By Name(cluster=w270, "Logging State"=enum16{"Configure", "Logging"}."Configure") -> (w268:T7)
        n104 = call <vilib>:"Add State(s) to Queue__JKI_lib_State_Machine.vi"("State(s) in Front (\"\")"="UI: Toggle Logging State\nXNETLog: Global Stop >> TRUE" ("State(s) in Front (\"\")"), "State(s) in (\"\")"=w273) -> ("States Out"=w272:string)  [unwired: 13 in]
      }
      frame "Macro: Exit" {
        # "Exit Macro\n(This is called once, when the VI exits)"
        n105 = Unbundle By Name(w280) -> ("Core.Close Panel on Exit?"=w279:bool)
        n106 = Select(t="UI: Front Panel State >> Close", s=w279, f="") -> (s? t:f=w276:string)
        n107 = call <vilib>:"Add State(s) to Queue__JKI_lib_State_Machine.vi"("State(s) in (\"\")"=w276, "State(s) at Back (\"\")"="Data: Cleanup\n\nMacro: Stop Logging\nError: Release Data Queue\n\nExit") -> ("States Out"=w274:string)  [unwired: 13 in]
        n108 = call <vilib>:"Add State(s) to Queue__JKI_lib_State_Machine.vi"("State(s) in Front (\"\")"=w274, "State(s) in (\"\")"=w283) -> ("States Out"=w282:string)  [unwired: 13 in]
      }
      frame "---------- Error ----------" {
        # "Template Separator\n(You can make a copy of, or modify, this frame)"
        n109 = call <vilib>:"Add State(s) to Queue__JKI_lib_State_Machine.vi"("State(s) in (\"\")"=w287) -> ("States Out"=w286:string)  [unwired: 14 in]
      }
      frame "Error: Obtain Error Queue" {
        n110 = global read "Global Variables.vi" "Error Queue Name"() -> (w292:string)
        n111 = Obtain Queue(name (unnamed)=w292, element data type=w289, error in (no error)=w289) -> (queue out=w288:refnum<queue>, error out=w291:errorcluster)  [unwired: 2 in, 1 out]
        n112 = Bundle By Name(cluster=w293, "Error Queue Ref"=w288) -> (w290:T7)
        n113 = call <vilib>:"Add State(s) to Queue__JKI_lib_State_Machine.vi"("State(s) in (\"\")"=w295) -> ("States Out"=w294:string)  [unwired: 14 in]
      }
      frame "Error: Release Data Queue" {
        n114 = Unbundle By Name(w299) -> ("Error Queue Ref"=w298:refnum<queue>)
        n115 = Release Queue(queue=w298, error in (no error)=w297) -> (error out=w296:errorcluster)  [unwired: 1 in, 2 out]
        n116 = call <vilib>:"Add State(s) to Queue__JKI_lib_State_Machine.vi"("State(s) in (\"\")"=w301) -> ("States Out"=w300:string)  [unwired: 14 in]
      }
      frame "Error: Handler" {
        n117 = Unbundle By Name(w308) -> ("Error Queue Ref"=w307:refnum<queue>)
        n118 = Dequeue Element(queue=w307, timeout in ms (-1)=0, error in (no error)=w306) -> (element=w302:errorcluster, error out=w305:errorcluster)  [unwired: 2 out]
        n119 = Merge Errors(w302, w305) -> (w303:errorcluster)
        n120 = call <vilib>:"Add State(s) to Queue__JKI_lib_State_Machine.vi"("State(s) in (\"\")"=w310) -> ("States Out"=w309:string)  [unwired: 14 in]
      }
      frame "---------- XNETLog ----------" {
        # "Template Separator\n(You can make a copy of, or modify, this frame)"
        n121 = call <vilib>:"Add State(s) to Queue__JKI_lib_State_Machine.vi"("State(s) in (\"\")"=w314) -> ("States Out"=w313:string)  [unwired: 14 in]
      }
      frame "XNETLog: Obtain Data Queue" {
        n122 = global read "Global Variables.vi" "XNET Data Queue Name"() -> (w320:string)
        n123 = Obtain Queue(name (unnamed)=w320, element data type=T5 {"PackageID"=0, "Data"=[]} ("Data Queue Type"), error in (no error)=w318) -> (queue out=w315:refnum<queue>, error out=w317:errorcluster)  [unwired: 2 in, 1 out]
        n124 = Bundle By Name(cluster=w321, "Data Queue Ref"=w315) -> (w316:T7)
        n125 = call <vilib>:"Add State(s) to Queue__JKI_lib_State_Machine.vi"("State(s) in (\"\")"=w323) -> ("States Out"=w322:string)  [unwired: 14 in]
      }
      frame "XNETLog: Release Data Queue" {
        n126 = Unbundle By Name(w327) -> ("Data Queue Ref"=w326:T6)
        n127 = Release Queue(queue=w326, error in (no error)=w325) -> (error out=w324:errorcluster)  [unwired: 1 in, 2 out]
        n128 = call <vilib>:"Add State(s) to Queue__JKI_lib_State_Machine.vi"("State(s) in (\"\")"=w329) -> ("States Out"=w328:string)  [unwired: 14 in]
      }
      frame "XNETLog: Check Data Queue State" {
        n129 = Unbundle By Name(w334) -> ("Data Queue Ref"=w333:T6)
        n130 = Get Queue Status(queue=w333, error in (no error)=w332) -> (error out=w331:errorcluster, # elements in queue=→"# elements in queue:":i32)  [unwired: 1 in, 6 out]
        n131 = call <vilib>:"Add State(s) to Queue__JKI_lib_State_Machine.vi"("State(s) in (\"\")"=w336) -> ("States Out"=w335:string)  [unwired: 14 in]
      }
      frame "XNETLog: Launch TDMS Writer" {
        n132 = Unbundle By Name(w342) -> ("LogFilePath"=w341:path, "CAN Configurations"=w338:refnum<vi>)
        n133 = property class="Arr (strict)"(reference=w338) -> ("Value"=w337:T1[])  [unwired: 1 in, 2 out]
        n134 = call "Launch Action - TDMS Writer.vi"("error in (no error)"=w340, "CAN Configurations"=w337, "Log file path"=w341) -> ("error out"=w339:errorcluster)  [unwired: 8 in]
        n135 = call <vilib>:"Add State(s) to Queue__JKI_lib_State_Machine.vi"("State(s) in (\"\")"=w344) -> ("States Out"=w343:string)  [unwired: 14 in]
      }
      frame "XNETLog: Launch XNET CAN Reader" {
        n136 = Unbundle By Name(w349) -> ("CAN Configurations"=w346:refnum<vi>)
        n137 = property class="Arr (strict)"(reference=w346) -> ("Value"=w345:T1[])  [unwired: 1 in, 2 out]
        n138 = call "Launch Action - XNET CAN Readers.vi"("error in (no error)"=w348, "CAN Configurations"=w345) -> ("error out"=w347:errorcluster)  [unwired: 9 in]
        n139 = call <vilib>:"Add State(s) to Queue__JKI_lib_State_Machine.vi"("State(s) in (\"\")"=w351) -> ("States Out"=w350:string)  [unwired: 14 in]
      }
      frame "XNETLog: Global Stop" {
        # "Template Separator\n(You can make a copy of, or modify, this frame)"
        n140 = case shown="\"False\", Default" w353 {
          tunnel: [_ TRUE ("Global Stop")] -> w352
          frame "False", Default {
          }
          frame "True" {
          }
        }
        n141 = global write "Global Variables.vi" "Global Stop"(w352) -> ()
        n142 = call <vilib>:"Add State(s) to Queue__JKI_lib_State_Machine.vi"("State(s) in (\"\")"=w357) -> ("States Out"=w356:string)  [unwired: 14 in]
      }
      frame "---------- Monitor ----------" {
        # "Template Separator\n(You can make a copy of, or modify, this frame)"
        n143 = call <vilib>:"Add State(s) to Queue__JKI_lib_State_Machine.vi"("State(s) in (\"\")"=w362) -> ("States Out"=w361:string)  [unwired: 14 in]
      }
      frame "Monitor: Initialize" {
        n144 = Unbundle By Name(w374) -> ("CAN Configurations"=w373:refnum<vi>)
        n145 = property class="Arr (strict)"(reference=w373) -> ("Value"=w372:T1[])  [unwired: 1 in, 2 out]
        n146 = call "Get Signal Names All.vi"("error in"=w370) -> ("error out"=w375:errorcluster, "Signal Names"=w369:string[])  [unwired: 9 in]
        n147 = To Variant(anything=waveform(dbl)[] [] ("Data")) -> (Variant=w365:variant)
        n148 = Array Size(array=w372) -> (size(s)=w367:i32)
        n149 = property on="Combo Box" class="CmbBox"("Strings[]"=w369) -> ()  [unwired: 2 in, 2 out]
        n150 = Initialize Array(w365, w367) -> (w364:variant[])
        n151 = call "Get Signal Units All.vi"("error in"=w375) -> ("error out"=w363:errorcluster, "Signal Units"=w368:string[])  [unwired: 9 in]
        n152 = global write "Global Variables.vi" "Signal Data"(w364) -> ()
        n153 = Bundle By Name(cluster=w374, "Monitor.SignalNames"=w369, "Monitor.SignalUnits"=w368) -> (w371:T7)
        n154 = call <vilib>:"Add State(s) to Queue__JKI_lib_State_Machine.vi"("State(s) in (\"\")"=w377) -> ("States Out"=w376:string)  [unwired: 14 in]
      }
      frame "Monitor: Update" {
        n155 = Unbundle By Name(w384) -> ("Monitor.SignalNames"=w383:string[])
        n156 = Unbundle By Name(w384) -> ("Monitor.SignalUnits"=w380:string[])
        n157 = call "Get Signal Data All.vi"("error in"=w386) -> ("error out"=w385:errorcluster, "Signal Data"=w381:waveform(dbl)[])  [unwired: 9 in]
        n158 = for {
          tunnel: w383 -> [w397]
          tunnel: "Monitor.SignalNames" -> [w396] mode=indexing
          tunnel: w381 -> [w395]
          tunnel: w380 -> [w394]
          tunnel: [w390] -> w379 mode=indexing
          tunnel: [w389] -> w378 mode=indexing
          n159 = Search 1D Array(1D array=w397, element=w396) -> (index of element=w393:i32)  [unwired: 1 in]
          n160 = Index Array(array=w395, index=w393) -> (element=w392:waveform(dbl))
          n161 = Index Array(array=w394, index=w393) -> (element=w389:string)
          n162 = Unbundle By Name(w392) -> ("Y"=w391:dbl[])
          n163 = Index Array(array=w391) -> (element=w390:dbl)  [unwired: 1 in]
        }
        "Monitor.SignalValues" <- w379
        "Monitor.SignalUnits" <- w378
        n164 = call <vilib>:"Add State(s) to Queue__JKI_lib_State_Machine.vi"("State(s) in (\"\")"=w388) -> ("States Out"=w387:string)  [unwired: 14 in]
      }
    }
  }
